vi "AutoCal.vi"() -> ()   [LabVIEW 2011]
panel:
  out "Distance Change":dbl
  out "Right Adj":dbl
  in  "Calibrate":bool
  in  "Distance":dbl=16.8
  in  "X2":dbl
  in  "X1":dbl
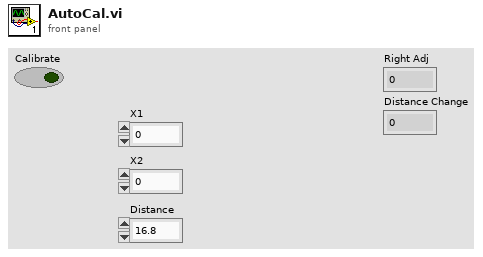
[diagram p1: front panel]
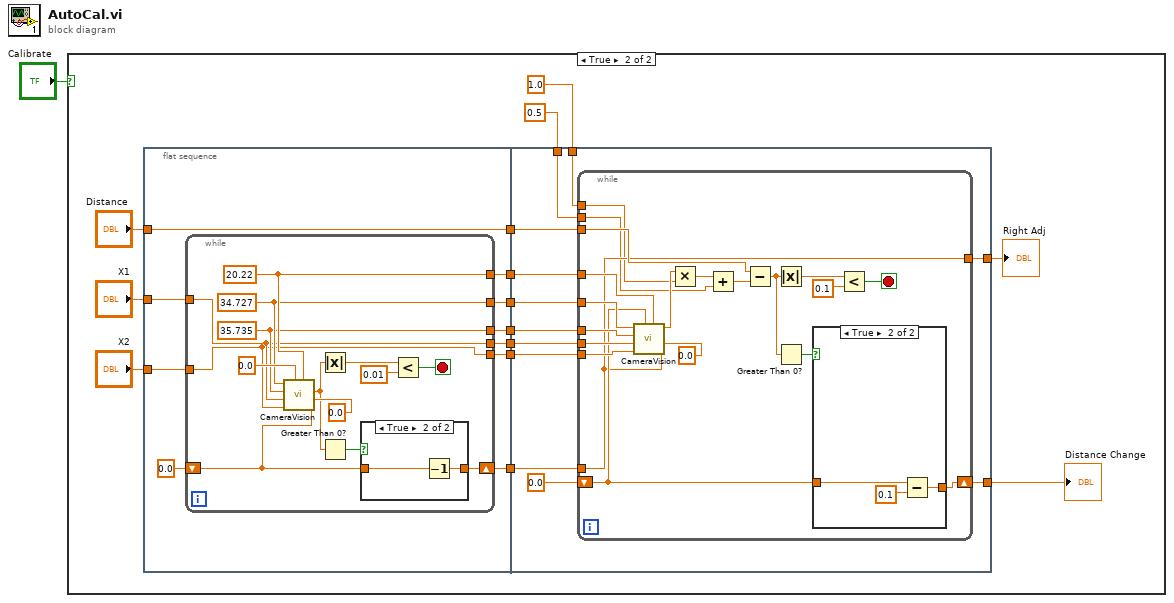
[diagram p0: block diagram]
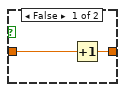
[diagram p3: hidden frame]
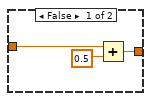
[diagram p4: hidden frame]
diagram:
  n1 = case shown="True" "Calibrate" {
    frame False {
    }
    frame True {
      n2 = flat-sequence {
        tunnel: "X1" -> [w25]
        tunnel: "X2" -> [w24]
        tunnel: "Distance" -> [w16]
        tunnel: [w22] -> w12
        tunnel: [w21] -> w11
        tunnel: [w20] -> w10
        tunnel: [w19] -> w9
        tunnel: [w18] -> w8
        tunnel: [w17] -> w7
        tunnel: [w16] -> w6
        tunnel: w12 -> [w55]
        tunnel: w11 -> [w54]
        tunnel: w10 -> [w53]
        tunnel: w9 -> [w52]
        tunnel: w8 -> [w50]
        tunnel: w7 -> [w49]
        tunnel: w6 -> [w48]
        tunnel: [w47] -> w5
        tunnel: [w46] -> w4
        tunnel: 1.0 ("y") -> [w45]
        tunnel: 0.5 ("y") -> [w44]
        frame #0 {
          n3 = while {
            tunnel: w25 -> [w27]
            tunnel: w24 -> [w26]
            shift-right: [w31] -> w22
            shift-left: 0.0 ("Distance Change") -> [w32]
            tunnel: [w30] -> w21
            tunnel: [w29] -> w20
            tunnel: [w28] -> w19
            tunnel: [w27] -> w18
            tunnel: [w26] -> w17
            stop <- w35 stop-if-true
            w30 = 20.22 ("W")
            w28 = 35.735 ("Left FOV")
            w29 = 34.727 ("Right FOV")
            n4 = call "CameraVision.vi"("X2 Change"=w32, "X1 Change"=0.0, "W"=w30, "Distance Change"=0.0, "x2"=w26, "x"=w27, "Left FOV"=w28, "Right FOV"=w29) -> ("Angle to Target"=w34:dbl)  [unwired: 1 in, 1 out]
            n5 = Absolute Value(x=w34) -> (abs(x)=w37:dbl)
            n6 = Greater Than 0?(x=w34) -> (x > 0?=w33:bool)
            n7 = case shown="True" w33 {
              tunnel: w32 -> [w41 w43]
              tunnel: [w40 w42] -> w31
              frame False {
                n8 = Increment(x=w41) -> (x+1=w40:dbl)
              }
              frame True {
                n9 = Decrement(x=w43) -> (x-1=w42:dbl)
              }
            }
            n10 = Less?(x=w37, y=0.01) -> (x < y?=w35:bool)
          }
        }
        frame #1 {
          n11 = while {
            tunnel: w55 -> [w61]
            tunnel: w54 -> [w71]
            tunnel: w53 -> [w70]
            tunnel: w52 -> [w69]
            shift-right: [w65] -> w46
            shift-left: 0.0 ("Distance Change") -> [w66]
            tunnel: w50 -> [w68]
            tunnel: w49 -> [w67]
            tunnel: w48 -> [w64]
            tunnel: [w61] -> w47
            tunnel: w45 -> [w57]
            tunnel: w44 -> [w56]
            stop <- w72 stop-if-true
            n12 = call "CameraVision.vi"("X2 Change"=w61, "X1 Change"=0.0, "W"=w71, "Distance Change"=w66, "x2"=w67, "x"=w68, "Left FOV"=w69, "Right FOV"=w70) -> ("Distance to Target"=w60:dbl)  [unwired: 1 in, 1 out]
            n13 = Multiply(x=w60, y=w57) -> (x*y=w59:dbl)
            n14 = Add(x=w59, y=w56) -> (x+y=w58:dbl)
            n15 = Subtract(x=w64, y=w58) -> (x-y=w63:dbl)
            n16 = Absolute Value(x=w63) -> (abs(x)=w74:dbl)
            n17 = Greater Than 0?(x=w63) -> (x > 0?=w62:bool)
            n18 = case shown="True" w62 {
              tunnel: w66 -> [w78 w81]
              tunnel: [w76 w79] -> w65
              frame False {
                n19 = Add(x=w78, y=0.5) -> (x+y=w76:dbl)
              }
              frame True {
                n20 = Subtract(x=w81, y=0.1) -> (x-y=w79:dbl)
              }
            }
            n21 = Less?(x=w74, y=0.1) -> (x < y?=w72:bool)
          }
        }
      }
      "Right Adj" <- w5
      "Distance Change" <- w4
    }
  }
